vi "FRCts20_Backend_EventRoot_GET.vi"(6 "Message Attributes":T4, 8 "error in (no error)":errorcluster, 10 "Data":string, 11 "Engine_Refnums":T1) -> (0 "error out":errorcluster)   [LabVIEW 2013, in "FRCts20_Backend_Engine.lvlib"]
doc: "Retrieves all event data, called by the Event Root API. Expects no input data."
uses:
  FRCts20_Backend_Engine.lvlib
  Dependencies/Keyed Array/KeyedArray.ctl
  FRCts20_Backend_EngineRefnums.ctl
  INI_Accessor/FRCts20_Backend_INI Controller.lvclass
  Dependencies/AMC/_SubVIs/TypeDefs/Message Queue.ctl
  Dependencies/AMC/_SubVIs/TypeDefs/Message.ctl
  <vilib>/addons/database/Connection.llb/Conn ObjectReference.ctl
  FRCts20_Backend_FGVOperation.ctl
  Dependencies/Keyed Array/Tools_KeyedArray.lvlib
  Dependencies/AMC/AMC.lvlib
  <vilib>/addons/database/NI_Database_API.lvlib
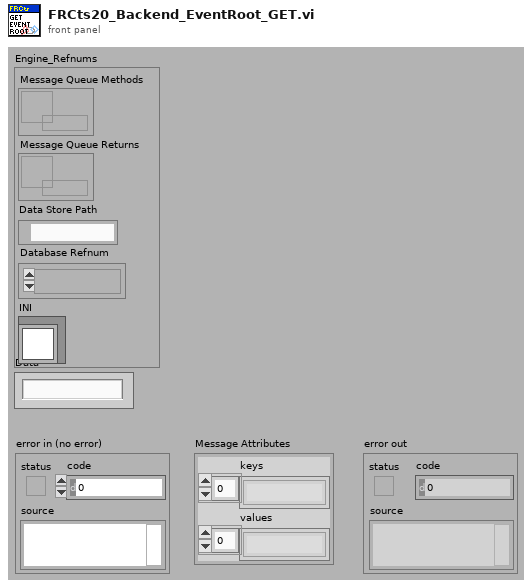
[diagram p1: front panel]
types:
  T1 = typedef "FRCts20_Backend_Engine.lvlib/FRCts20_Backend_EngineRefnums.ctl" = cluster{"Message Queue Methods":T2, "Message Queue Returns":T2, "Data Store Path":path, "Database Refnum":T3, "INI":refnum<class "FRCts20_Backend_INI Controller.lvclass">}
  T2 = typedef "AMC.lvlib/Message Queue.ctl" = refnum<queue>
  T3 = typedef "NI_Database_API.lvlib/Conn ObjectReference.ctl" = refnum<k1>
  T4 = typedef "Tools_KeyedArray.lvlib/KeyedArray.ctl" = cluster{"keys":string[], "values":string[]}
  T5 = typedef "FRCts20_Backend_Engine.lvlib/FRCts20_Backend_FGVOperation.ctl" = enum16{"Initialize", "EnqueueMessage", "EnqueueDataReturn", "FlushMessage", "FlushDataReturn"}
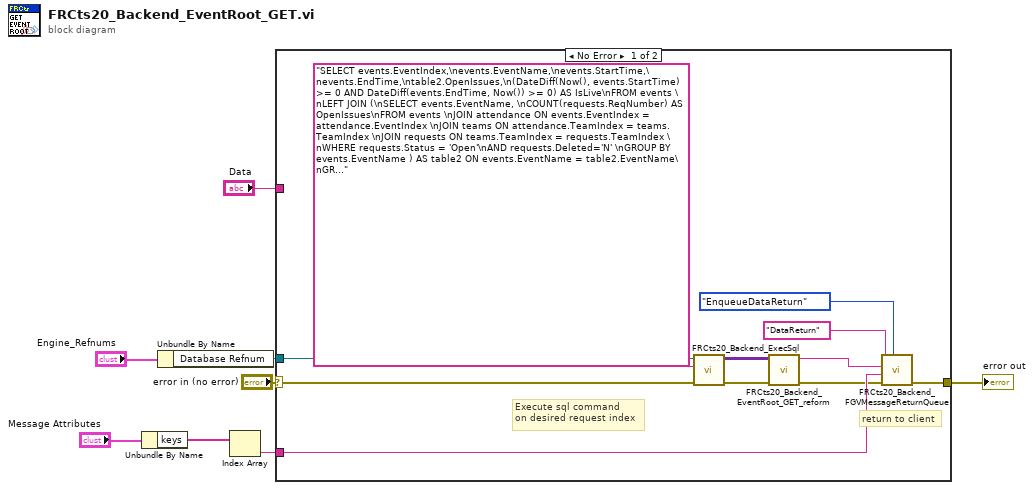
[diagram p0: block diagram]
diagram:
  n1 = Unbundle By Name("Message Attributes") -> ("keys"=w4:string[])
  n2 = Unbundle By Name("Engine_Refnums") -> ("Database Refnum"=w1:T3)
  n3 = Index Array(array=w4) -> (element=w3:string)  [unwired: 1 in]
  n4 = case shown="No Error" "error in (no error)" {
    selector: "error in (no error)" -> [w11 w20]
    tunnel: [w19 w20] -> w7
    tunnel: w1 -> [w12 _]
    tunnel: "Data" -> [_ _]
    tunnel: w3 -> [w18 _]
    frame No Error {
      # "return to client"
      # "Execute sql command\non desired request index"
      n5 = call "FRCts20_Backend_ExecSql.vi"("error in (no error)"=w11, "format string"="SELECT events.EventIndex,\nevents.EventName,\nevents.StartTime,\nevents.EndTime,\ntable2.OpenIssues,\n(DateDiff(Now(), events.StartTime) >= 0 AND DateDiff(events.EndTime, Now()) >= 0) AS IsLive\nFROM events \nLEFT JOIN (\nSELECT events.EventName, \nCOUNT(requests.ReqNumber) AS OpenIssues\nFROM events \nJOIN attendance ON events.EventIndex = attendance.EventIndex \nJOIN teams ON attendance.TeamIndex = teams.TeamIndex \nJOIN requests ON teams.TeamIndex = requests.TeamIndex \nWHERE requests.Status = 'Open'\nAND requests.Deleted='N' \nGROUP BY events.EventName ) AS table2 ON events.EventName = table2.EventName\nGROUP BY events.EventIndex", "Refnum in"=w12) -> ("error out"=w17:errorcluster, "recordset data"=w9:variant[][])  [unwired: 6 in, 1 out]
      n6 = call "FRCts20_Backend_EventRoot_GET_reform.vi"("error in (no error)"=w17, "recordset data"=w9) -> ("error out"=w13:errorcluster, "data string"=w14:string)  [unwired: 8 in]
      n7 = call "FRCts20_Backend_FGVMessageReturnQueue.vi"("Operation"=FRCts20_Backend_FGVOperation."EnqueueDataReturn", "error in (no error)"=w13, "Key"=w18, "Message Value"=w14, "Message Name"="DataReturn") -> ("error out"=w19:errorcluster)  [unwired: 5 in, 1 out]
    }
    frame Error {
    }
  }
  "error out" <- w7
